vi "Do Flash.vi"(10 "x > y?":bool[][](array[boolean]), 11 "Octopus Energy Levels in":i32[][](array[numeric])) -> (2 "No of flashes":i32, 3 "Octopus Energy Levels out":i32[][](array[numeric]))   [LabVIEW 2021]
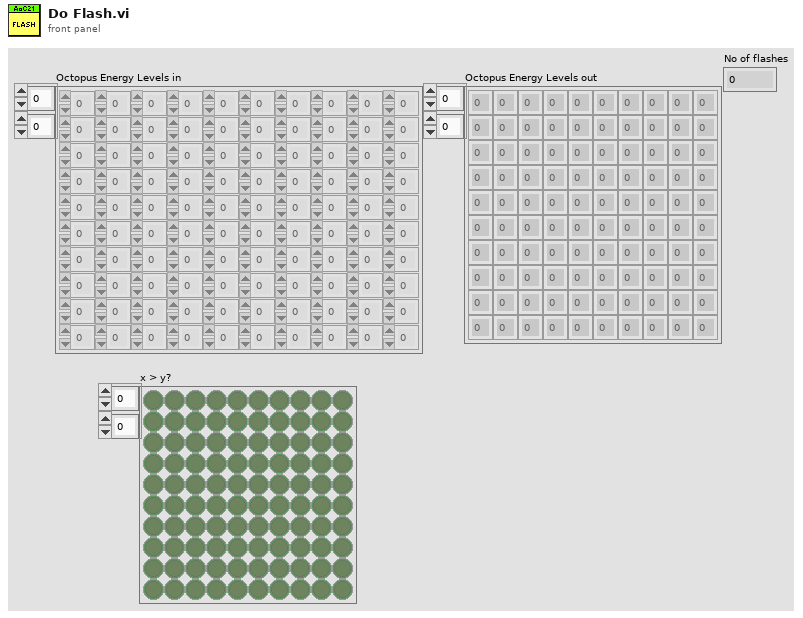
[diagram p1: front panel]
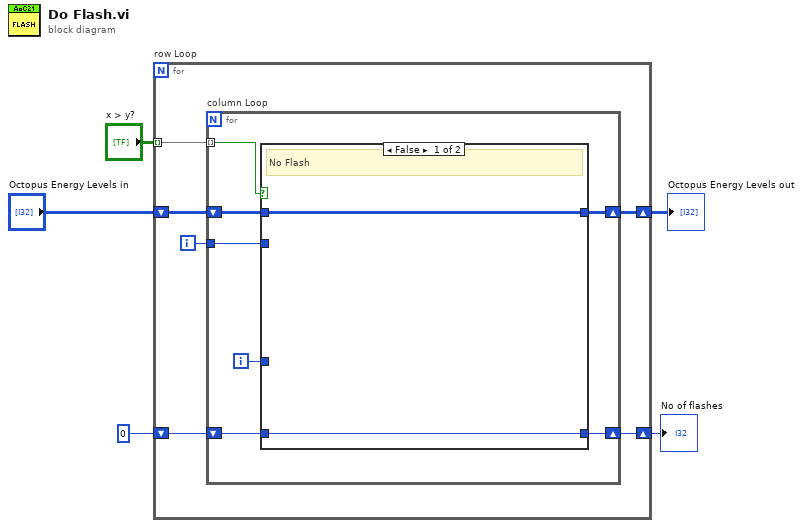
[diagram p0: block diagram]
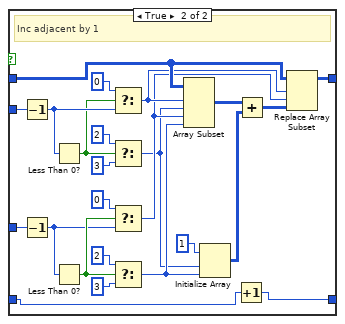
[diagram p2: hidden frame]
diagram:
  n1 = for "row Loop" {
    tunnel: "x > y?" -> [w11] mode=indexing
    shift-right: [w9] -> w3
    shift-left: "Octopus Energy Levels in" -> [w10]
    shift-right: [w6] -> w1
    shift-left: 0 -> [w7]
    i -> [w8]
    n2 = for "column Loop" {
      tunnel: w11 -> [w18] mode=indexing
      shift-right: [w16] -> w9
      shift-left: w10 -> [w17]
      tunnel: w8 -> [w14]
      shift-right: [w12] -> w6
      shift-left: w7 -> [w13]
      i -> [w15]
      n3 = case shown="False" w18 {
        tunnel: [w20 w40] -> w16
        tunnel: w17 -> [w20 w39]
        tunnel: w15 -> [_ w41]
        tunnel: w14 -> [_ w42]
        tunnel: w13 -> [w19 w22]
        tunnel: [w19 w21] -> w12
        frame False {
          # "No Flash"
        }
        frame True {
          # "Inc adjacent by 1"
          n4 = Decrement(x=w42) -> (x-1=w36:i32)
          n5 = Decrement(x=w41) -> (x-1=w27:i32)
          n6 = Less Than 0?(x=w36) -> (x < 0?=w34:bool)
          n7 = Less Than 0?(x=w27) -> (x < 0?=w29:bool)
          n8 = Select(t=0, s=w34, f=w36) -> (s? t:f=w26:i32)
          n9 = Select(t=2 ("dimension size"), s=w34, f=3 ("dimension size")) -> (s? t:f=w23:i32)
          n10 = Select(t=0, s=w29, f=w27) -> (s? t:f=w25:i32)
          n11 = Select(t=2 ("dimension size"), s=w29, f=3 ("dimension size")) -> (s? t:f=w24:i32)
          n12 = Array Subset(array=w39, index (row)=w26, length (row)=w23, index (col)=w25, length (col)=w24) -> (w37:i32[][])
          n13 = Initialize Array(1, w23, w24) -> (w43:i32[][])
          n14 = Increment(x=w22) -> (x+1=w21:i32)
          n15 = Add(x=w37, y=w43) -> (x+y=w38:i32[][])
          n16 = Replace Array Subset(array=w39, new element=w38, index (row)=w26, index (col)=w25) -> (w40:i32[][])
        }
      }
    }
  }
  "Octopus Energy Levels out" <- w3
  "No of flashes" <- w1
